vi "Send_Classification.vi"(0 "logging FIFO":refnum<k33>, 1 "Classification FIFO":refnum<k33>, 2 "Window":sgl[][](array[numeric]), 3 "error in (no error)":errorcluster) -> (6 "Sended frame":dbl[](array[numeric]))   [LabVIEW 2020]
uses:
  Global Variables/Global Enable Logging.vi
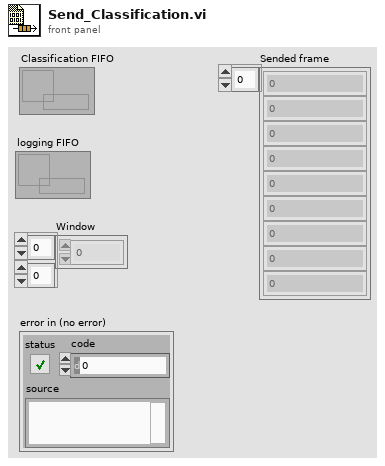
[diagram p1: front panel]
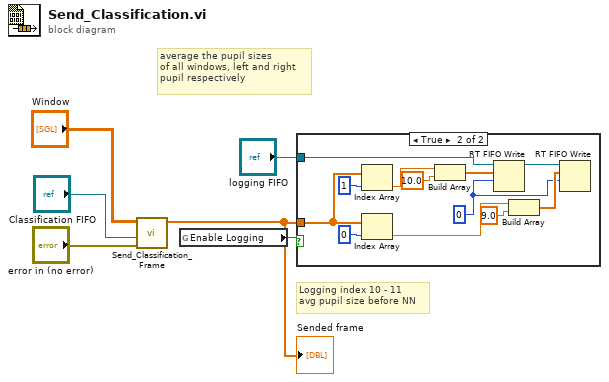
[diagram p0: block diagram]
diagram:
  # "Logging index 10 - 11 \navg pupil size before NN"
  # "average the pupil sizes \nof all windows, left and right\npupil respectively"
  n1 = call "Send_Classification_Frame.vi"("error in (no error)"="error in (no error)", "rt fifo single"="Classification FIFO", "Pre-Partition"="Window") -> ("Sended frame"=w5:dbl[])  [unwired: 4 in, 1 out]
  "Sended frame" <- w5
  n2 = global read "Global Enable Logging.vi" "Enable Logging"() -> (w6:bool)
  n3 = case shown="True" w6 {
    tunnel: "logging FIFO" -> [_ w18]
    tunnel: w5 -> [_ w15]
    frame False {
    }
    frame True {
      w7 = 0 ("timeout in ms (0)")
      n4 = Index Array(array=w15, index=1) -> (element=w13:dbl)
      n5 = Index Array(array=w15, index=0) -> (element=w11:dbl)
      n6 = Build Array(w13, 10.0 ("element")) -> (w10:dbl[])
      n7 = RT FIFO Write(0:w18, 1:w10, 2:w7) -> (8:w9:refnum<k33>)  [unwired: 2 in, 3 out]
      n8 = Build Array(w11, 9.0 ("element")) -> (w8:dbl[])
      n9 = RT FIFO Write(0:w9, 1:w8, 2:w7) -> ()  [unwired: 2 in, 4 out]
    }
  }
